vi "cmc_inclass_tempconversion.vi"(8 "error in (no error)":errorcluster, 10 "Desired Temperature\nMeasure":T1(ring), 11 "Type K Voltage(V)":dbl) -> (0 "error out":errorcluster, 2 "Temperature\nMeasure":T1(ring), 3 "Temperature":dbl)   [LabVIEW 2010]
doc: "This VI will take a type K voltage in volts and covert to temperature based on the data provided by the manufacturer. There is also the option of converting to different measures of temperature besides Celsius. And any error will result in NaN being displayed in the temperature\n\nRochester Institute of Technology\nMechanical Engineering Department\nClair Cunningham"
panel:
  out "High":dbl[](array[numeric])
  out "Mid":dbl[](array[numeric])
  out "Low":dbl[](array[numeric])
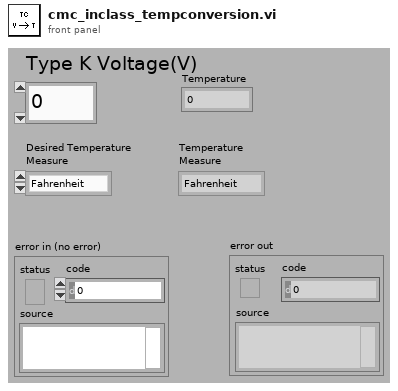
[diagram p1: front panel]
types:
  T1 = enum16{"Fahrenheit", "Celsius", "Kelvin", "Rankine"}
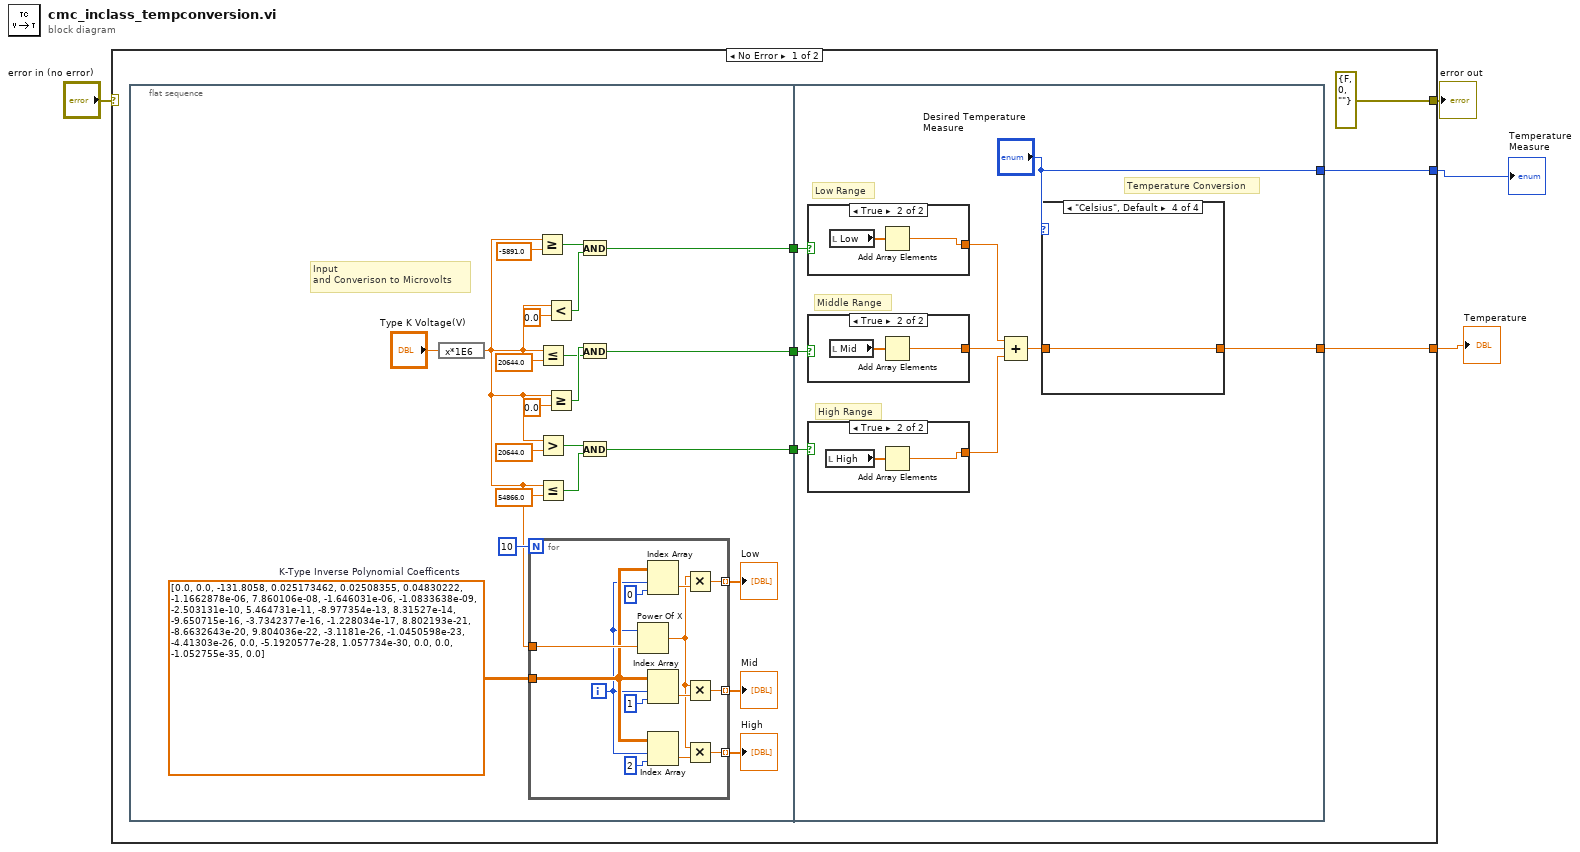
[diagram p0: block diagram]
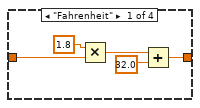
[diagram p2: hidden frame]
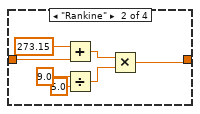
[diagram p3: hidden frame]
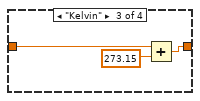
[diagram p4: hidden frame]
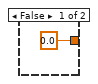
[diagram p5: hidden frame]
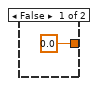
[diagram p6: hidden frame]
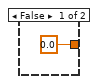
[diagram p7: hidden frame]
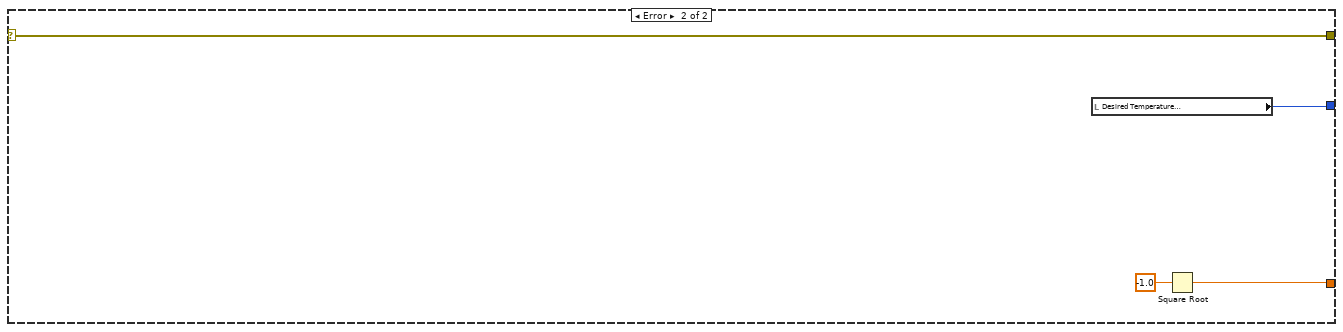
[diagram p8: hidden frame]
diagram:
  n1 = case shown="No Error" "error in (no error)" {
    selector: "error in (no error)" -> [_ w83]
    tunnel: [errorcluster {"status"=FALSE, "code"=0, "source"=""} ("error IO") w83] -> w3
    tunnel: [w6 w82] -> w2
    tunnel: [w5 w80] -> w1
    frame No Error {
      n2 = flat-sequence {
        tunnel: [w25] -> w10
        tunnel: [w24] -> w9
        tunnel: [w17] -> w8
        tunnel: w10 -> [w50]
        tunnel: w9 -> [w51]
        tunnel: w8 -> [w49]
        tunnel: [w47] -> w6
        tunnel: ["Desired Temperature\nMeasure"] -> w5
        frame #0 {
          w14 = dbl[][] [[0.0, 0.0, -131.8058], [0.025173462, 0.02508355, 0.04830222], [-1.1662878e-06, 7.860106e-08, -1.646031e-06], [-1.0833638e-09, -2.503131e-10, 5.464731e-11], [-8.977354e-13, 8.31527e-14, -9.650715e-16], [-3.7342377e-16, -1.228034e-17, 8.802193e-21], [-8.6632643e-20, 9.804036e-22, -3.1181e-26], [-1.0450598e-23, -4.41303e-26, 0.0], [-5.1920577e-28, 1.057734e-30, 0.0], [0.0, -1.052755e-35, 0.0]]  # K-Type Inverse Polynomial Coefficents
          # "Input \nand Converison to Microvolts"
          n3 = expression code="x*1E6"("Type K Voltage(V)") -> (w15:dbl)
          n4 = for {
            N: 10 -> [_]
            tunnel: w15 -> [w45]
            tunnel: w14 -> [w37]
            tunnel: [w39] -> w13 mode=indexing
            tunnel: [w38] -> w12 mode=indexing
            tunnel: [w33] -> w11 mode=indexing
            i -> [w36]
            n5 = Power Of X(1:w45, 2:w36) -> (0:w35:dbl)
            n6 = Index Array(array=w37, index (row)=w36, index (col)=0 ("disabled index (col)")) -> (element=w42:dbl)
            n7 = Index Array(array=w37, index (row)=w36, index (col)=1 ("disabled index (col)")) -> (element=w41:dbl)
            n8 = Index Array(array=w37, index (row)=w36, index (col)=2 ("disabled index (col)")) -> (element=w34:dbl)
            n9 = Multiply(x=w35, y=w42) -> (x*y=w39:dbl)
            n10 = Multiply(x=w35, y=w41) -> (x*y=w38:dbl)
            n11 = Multiply(x=w35, y=w34) -> (x*y=w33:dbl)
          }
          "Low" <- w13
          "Mid" <- w12
          "High" <- w11
          n12 = Greater Or Equal?(x=w15, y=-5891.0) -> (x >= y?=w30:bool)
          n13 = Less Or Equal?(x=w15, y=20644.0) -> (x <= y?=w26:bool)
          n14 = Greater?(x=w15, y=20644.0) -> (0:w23:bool)
          n15 = Less Or Equal?(x=w15, y=54866.0) -> (x <= y?=w22:bool)
          n16 = Less?(x=w15, y=0.0) -> (x < y?=w29:bool)
          n17 = Greater Or Equal?(x=w15, y=0.0) -> (x >= y?=w27:bool)
          n18 = And(x=w30, y=w29) -> (x .and. y?=w17:bool)
          n19 = And(x=w27, y=w26) -> (x .and. y?=w25:bool)
          n20 = And(x=w23, y=w22) -> (x .and. y?=w24:bool)
        }
        frame #1 {
          # "Temperature Conversion"
          # "High Range"
          # "Middle Range"
          # "Low Range"
          n21 = case shown="True" w49 {
            tunnel: [0.0 w78] -> w52
            frame False {
            }
            frame True {
              n22 = local read "Low"() -> (w79:dbl[])
              n23 = Add Array Elements(numeric array=w79) -> (sum=w78:dbl)
            }
          }
          n24 = case shown="True" w50 {
            tunnel: [0.0 w75] -> w53
            frame False {
            }
            frame True {
              n25 = local read "Mid"() -> (w76:dbl[])
              n26 = Add Array Elements(numeric array=w76) -> (sum=w75:dbl)
            }
          }
          n27 = case shown="True" w51 {
            tunnel: [0.0 w72] -> w54
            frame False {
            }
            frame True {
              n28 = local read "High"() -> (w73:dbl[])
              n29 = Add Array Elements(numeric array=w73) -> (sum=w72:dbl)
            }
          }
          n30 = Compound Arithmetic op=ADD(w52, w53, w54) -> (w48:dbl)
          n31 = case shown="\"Celsius\", Default" "Desired Temperature\nMeasure" {
            tunnel: w48 -> [w59 w66 w68 w70]
            tunnel: [w55 w60 w67 w70] -> w47
            frame "Fahrenheit" {
              n32 = Multiply(x=1.8, y=w59) -> (x*y=w56:dbl)
              n33 = Add(x=w56, y=32.0) -> (x+y=w55:dbl)
            }
            frame "Rankine" {
              n34 = Add(x=273.15, y=w66) -> (x+y=w62:dbl)
              n35 = Divide(x=9.0, y=5.0) -> (x/y=w61:dbl)
              n36 = Multiply(x=w62, y=w61) -> (x*y=w60:dbl)
            }
            frame "Kelvin" {
              n37 = Add(x=w68, y=273.15) -> (x+y=w67:dbl)
            }
            frame "Celsius", Default {
            }
          }
        }
      }
    }
    frame Error {
      n38 = local read "Desired Temperature\nMeasure"() -> (w80:T1)
      n39 = Square Root(x=-1.0) -> (sqrt(x)=w82:dbl)
    }
  }
  "error out" <- w3
  "Temperature" <- w2
  "Temperature\nMeasure" <- w1
